vi "StateMachine.vi"   [LabVIEW 2020]
uses:
  States.ctl
types:
  T1 = typedef "States.ctl" = enum16{"Idle", "Initialize", "Process1", "Process2", "Exit"}
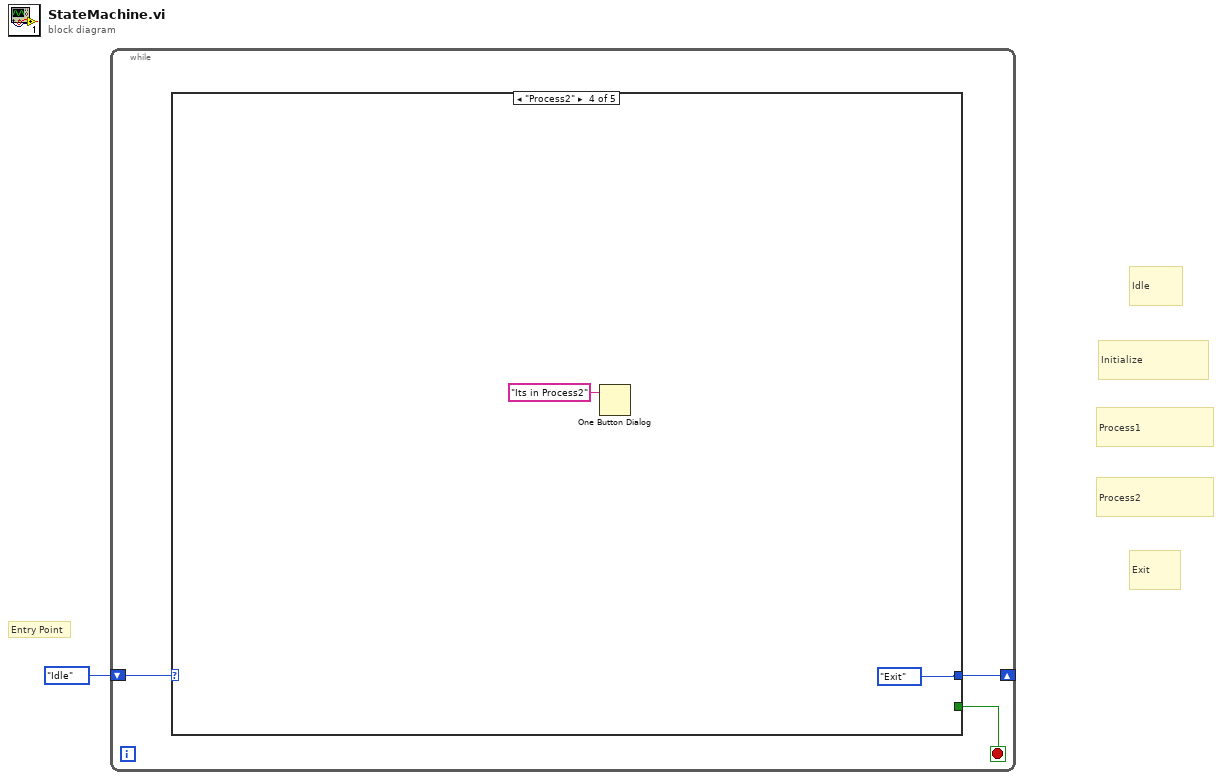
[diagram p0: block diagram]
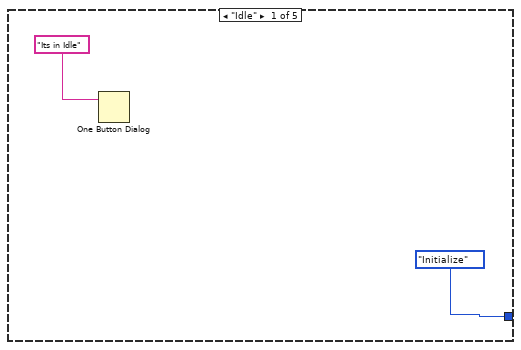
[diagram p2: hidden frame]
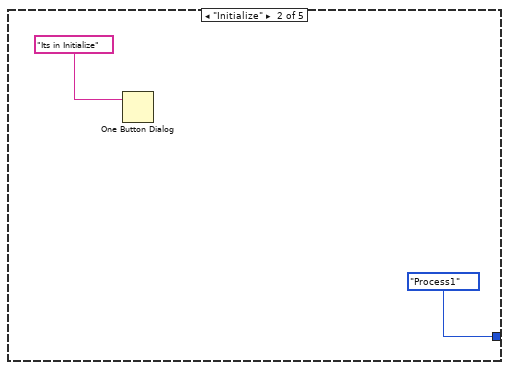
[diagram p3: hidden frame]
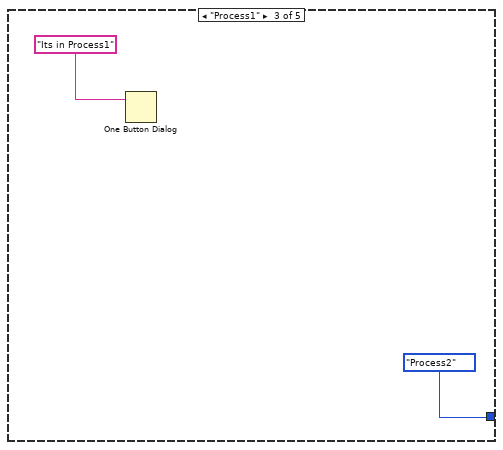
[diagram p4: hidden frame]
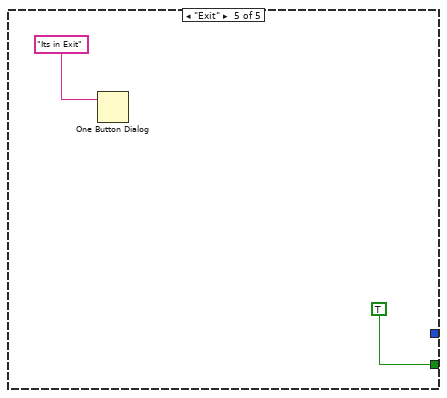
[diagram p5: hidden frame]
diagram:
  # "Entry Point"
  # "Idle"
  # "Exit"
  # "Process2"
  # "Process1"
  # "Initialize"
  n1 = while {
    shift-right: [w3] -> _
    shift-left: States."Idle" -> [w4]
    stop <- w2 stop-if-true
    n2 = case shown="\"Process2\"" w4 {
      tunnel: [States."Initialize" States."Process1" States."Process2" States."Exit" _] -> w3
      tunnel: [_ _ _ _ TRUE] -> w2
      frame "Idle" {
        n3 = One Button Dialog(message="Its in Idle") -> ()  [unwired: 1 in, 1 out]
      }
      frame "Initialize" {
        n4 = One Button Dialog(message="Its in Initialize") -> ()  [unwired: 1 in, 1 out]
      }
      frame "Process1" {
        n5 = One Button Dialog(message="Its in Process1") -> ()  [unwired: 1 in, 1 out]
      }
      frame "Process2" {
        n6 = One Button Dialog(message="Its in Process2") -> ()  [unwired: 1 in, 1 out]
      }
      frame "Exit" {
        n7 = One Button Dialog(message="Its in Exit") -> ()  [unwired: 1 in, 1 out]
      }
    }
  }
